vi "Write Object Name.vi"(8 "error in (no error)":errorcluster, 10 "Object Name":string, 11 "Base in":refnum<class "CS++Base.lvclass">) -> (0 "error out":errorcluster, 3 "Base out":refnum<class "CS++Base.lvclass">)   [LabVIEW 2012, in "CS++BaseClasses.lvlib" / "CS++Base.lvclass"]
doc: "Write name of object."
uses:
  CS++Base.lvclass
  CS++Base.lvclass/CS++Base.ctl
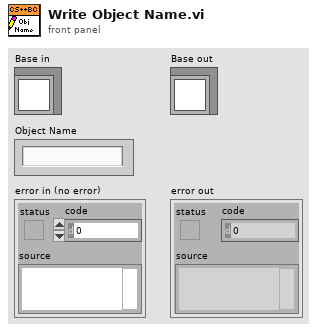
[diagram p1: front panel]
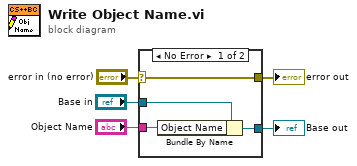
[diagram p0: block diagram]
diagram:
  n1 = case shown="No Error" "error in (no error)" {
    selector: "error in (no error)" -> [w9 w10]
    tunnel: [w9 w10] -> w4
    tunnel: [w7 w11] -> w2
    tunnel: "Base in" -> [w8 w11]
    tunnel: "Object Name" -> [w6 _]
    frame No Error {
      n2 = Bundle By Name(cluster=w8, "Object Name"=w6) -> (w7:refnum<class "CS++Base.lvclass">)
    }
    frame Error {
    }
  }
  "error out" <- w4
  "Base out" <- w2
